vi "Example2.1.vi"() -> ()   [LabVIEW 2019]
panel:
  out "Timer Done":bool
  in  "Wait Time (Seconds)":dbl=4.0
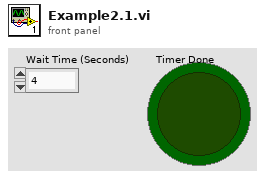
[diagram p1: front panel]
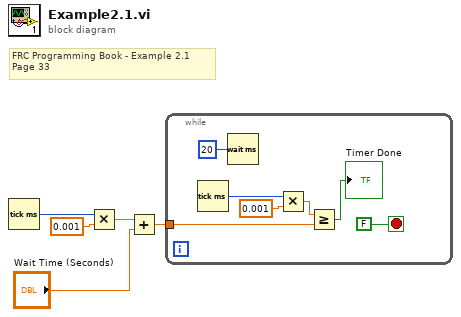
[diagram p0: block diagram]
diagram:
  # "FRC Programming Book - Example 2.1\nPage 33"
  n1 = Tick Count (ms)() -> (millisecond timer value=w4:u32)
  n2 = Multiply(x=w4, y=0.001) -> (x*y=w2:dbl)
  n3 = Add(x=w2, y="Wait Time (Seconds)") -> (x+y=w1:dbl)
  n4 = while {
    tunnel: w1 -> [w12]
    stop <- FALSE stop-if-true
    n5 = Tick Count (ms)() -> (millisecond timer value=w9:u32)
    n6 = Wait (ms)(milliseconds to wait=u32 20) -> ()  [unwired: 1 out]
    n7 = Multiply(x=w9, y=0.001) -> (x*y=w8:dbl)
    n8 = Greater Or Equal?(x=w8, y=w12) -> (x >= y?=→"Timer Done":bool)
  }
